vi "State Description - Helper VI and Equivalent String.vi"() -> ()   [LabVIEW 2014]
uses:
  user.lib/_NEVSTOP/JKI State Machine++/_Polymophic/Build No-Reply Asynchronous Message with Arguments.vi
  user.lib/_NEVSTOP/JKI State Machine++/_Polymophic/Build Asynchronous Message with Arguments.vi
  user.lib/_NEVSTOP/JKI State Machine++/_Polymophic/Build Synchronous Message with Arguments.vi
  user.lib/_NEVSTOP/JKI State Machine++/_Support/Message/Parse State with Arguments String.vi
  user.lib/_NEVSTOP/JKI State Machine++/JKI State Machine++.lvlib
panel:
  out "Equivalent String (Async without reply Message)":string="State >> Argument->DestModuleName"
  out "Equivalent String (Broadcast Message with Argument)":string="Status Changed >> Argument-> <all>"
  out "Equivalent String (Broadcast Message)":string="Status Changed-> <all>"
  out "Equivalent String (Async Message)":string="State >> Argument->DestModuleName"
  out "Equivalent String (Sync Message)":string="State >> Argument@DestModuleName"
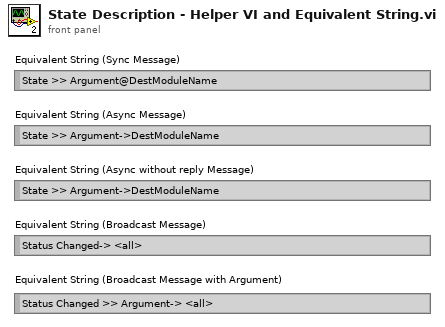
[diagram p1: front panel]
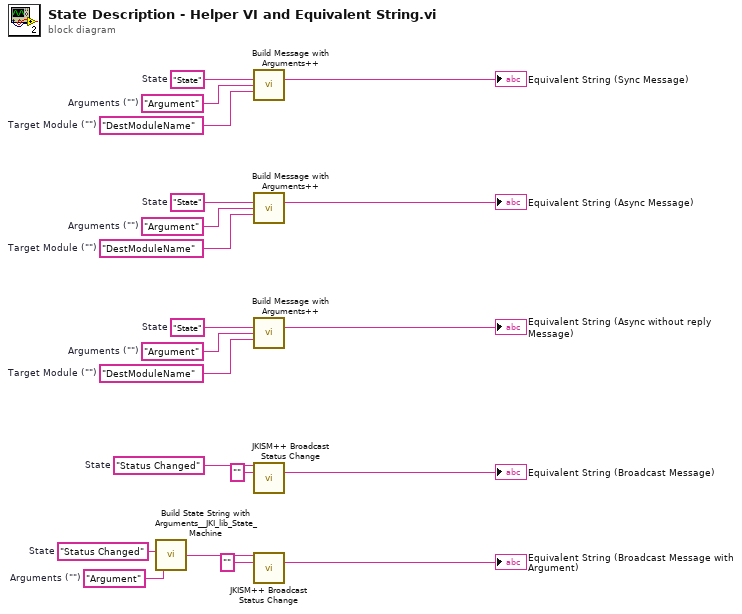
[diagram p0: block diagram]
diagram:
  w3 = "Argument"  # Arguments ("")
  w2 = "DestModuleName"  # Target Module ("")
  w4 = "State"  # State
  w7 = "Argument"  # Arguments ("")
  w6 = "Status Changed"  # State
  w12 = "Status Changed"  # State
  w14 = "Argument"  # Arguments ("")
  w15 = "DestModuleName"  # Target Module ("")
  w13 = "State"  # State
  w19 = "Argument"  # Arguments ("")
  w18 = "DestModuleName"  # Target Module ("")
  w20 = "State"  # State
  n1 = call <vilib>:"Build State String with Arguments__JKI_lib_State_Machine.vi"("Arguments (\"\")"=w7, "State"=w6) -> ("State with Arguments"=w5:string)  [unwired: 4 in]
  n2 = call-poly "Build Message with Arguments++.vi"("State with Arguments"=w20, "Arguments (\"\")"=w19, "Target Module (\"\")"=w18) -> ("State with Arguments"=→"Equivalent String (Sync Message)":string)  [unwired: 12 in]
  n3 = call-poly "Build Message with Arguments++.vi"("State with Arguments"=w13, "Arguments (\"\")"=w14, "Target Module (\"\")"=w15) -> ("State with Arguments"=→"Equivalent String (Async Message)":string)  [unwired: 12 in]
  n4 = call-poly "Build Message with Arguments++.vi"("State with Arguments"=w4, "Arguments (\"\")"=w3, "Target Module (\"\")"=w2) -> ("State with Arguments"=→"Equivalent String (Async without reply Message)":string)  [unwired: 12 in]
  n5 = call "JKISM++ Broadcast Status Change.vi"("Status with Arguments"=w12, "State Queue"="" ("State(s) in (\"\")")) -> ("Remaining States"=→"Equivalent String (Broadcast Message)":string)  [unwired: 13 in]
  n6 = call "JKISM++ Broadcast Status Change.vi"("Status with Arguments"=w5, "State Queue"="" ("State(s) in (\"\")")) -> ("Remaining States"=→"Equivalent String (Broadcast Message with Argument)":string)  [unwired: 13 in]
